vi "StatusQueryParser.vi"(11 "Numeric":i8) -> (3 "String":string)   [LabVIEW 2017, in "Fridge Software v2.1.lvlib"]
uses:
  Fridge Software v2.1.lvlib
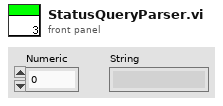
[diagram p1: front panel]
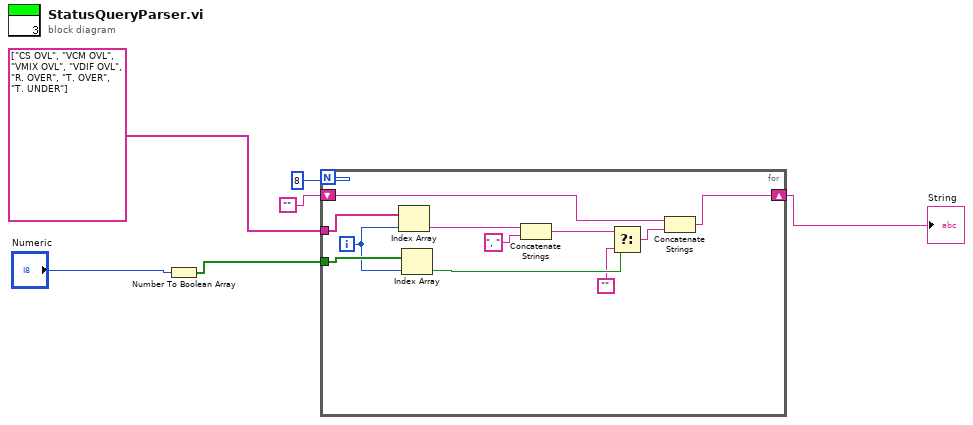
[diagram p0: block diagram]
diagram:
  n1 = Number To Boolean Array(number="Numeric") -> (Boolean array=w3:bool[])
  n2 = for {
    N: 8 -> [_]
    tunnel: string[] ["CS OVL", "VCM OVL", "VMIX OVL", "VDIF OVL", "R. OVER", "T. OVER", "T. UNDER"] -> [w17]
    tunnel: w3 -> [w16]
    shift-right: [w11] -> w2
    shift-left: "" -> [w9]
    i -> [w14]
    n3 = Index Array(array=w17, index=w14) -> (element=w12:string)
    n4 = Index Array(array=w16, index=w14) -> (element=w15:bool)
    n5 = Concatenate Strings(w12, ", ") -> (w8:string)
    n6 = Select(t=w8, s=w15, f="") -> (s? t:f=w10:string)
    n7 = Concatenate Strings(w9, w10) -> (w11:string)
  }
  "String" <- w2
